vi "CODMn手动控制框.vi"(8 "Error in":errorcluster, 11 "MB_Serial session":refnum<class "MB_Master_Serial.lvclass">) -> ()   [LabVIEW 2016, in "斯坦道CODMn.lvlib"]
uses:
  <vilib>/Plasmionique/MB Master/MB_Master_Serial/MB_Master_Serial.lvclass
  C:/Program Files (x86)/National Instruments/LabVIEW 2016/vi.lib/Plasmionique/MB Master/MB_Master/MB_Master.lvclass
  <vilib>/Plasmionique/MB Master/MB Master.lvlib
panel:
  in  "2#排":bool
  in  "2#进":bool
  in  "2#复位":bool
  in  "1#排":bool
  in  "1#进":bool
  in  "1#复位":bool
  in  "风扇":bool
  in  "排液":bool
  in  "搅拌":bool
  in  "加热":bool
  in  "硫酸":bool
  in  "加标回收样":bool
  in  "质控样":bool
  in  "标液":bool
  in  "纯水":bool
  in  "退出":bool
  in  "水样":bool
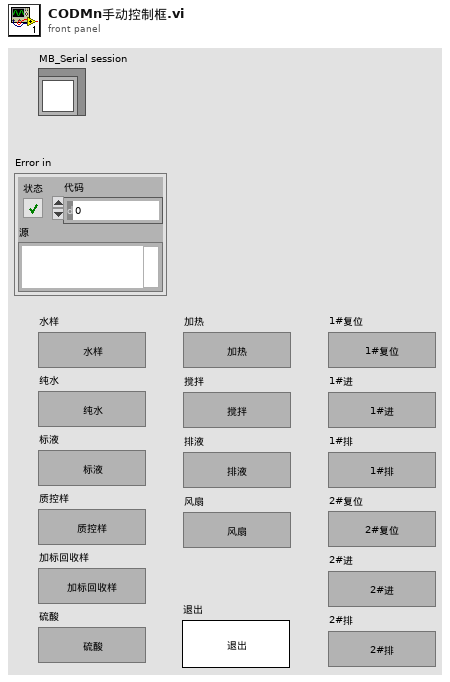
[diagram p1: front panel]
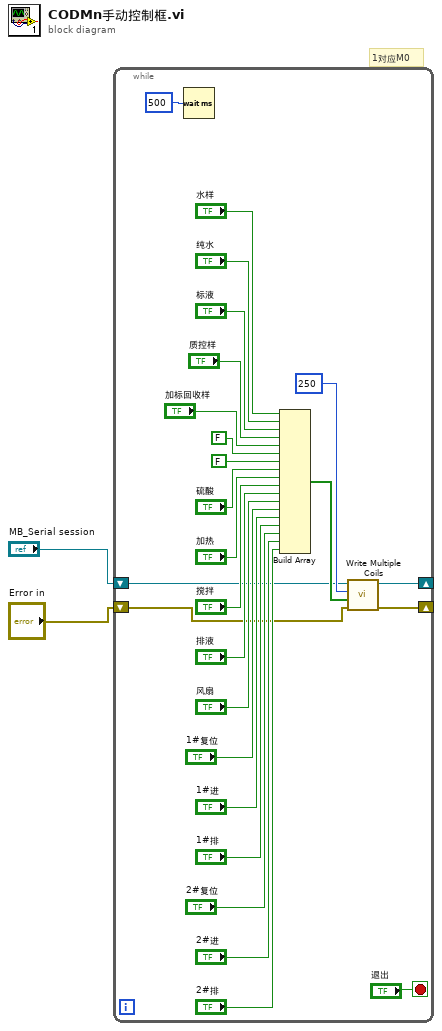
[diagram p0: block diagram]
diagram:
  # "1对应M0"
  n1 = while {
    shift-right: [w6] -> _
    shift-left: "MB_Serial session" -> [w4]
    shift-right: [w5] -> _
    shift-left: "Error in" -> [w3]
    stop <- "退出" stop-if-true
    n2 = Wait (ms)(milliseconds to wait=u32 500 ("等待时间（毫秒）")) -> ()  [unwired: 1 out]
    n3 = Build Array("水样", "纯水", "标液", "质控样", "加标回收样", FALSE ("元素"), FALSE ("元素"), "硫酸", "加热", "搅拌", "排液", "风扇", "1#复位", "1#进", "1#排", "2#复位", "2#进", "2#排") -> (w25:bool[])
    n4 = call <vilib>:"Write Multiple Coils.vi"("error in (no error)"=w3, "values"=w25, "starting address"=u16 250, "MB session in"=w4) -> ("error out"=w5:errorcluster, "MB session out"=w6:refnum<class "MB_Master_Serial.lvclass">)  [unwired: 6 in]
  }
